vi "Log Message with Level.vi"(6 "Log Level (INFO)":T1=enum."INFO", 8 "error in (no error)":errorcluster, 11 "Message":string) -> (0 "error out":errorcluster)   [LabVIEW 2020, in "RxnRover.lvlib" / "logging.lvlib"]
doc: "Log the given message to the Rxn Rover log file. Appends the log level, date, and time to the message."
uses:
  logging.lvlib
  Log Levels.ctl
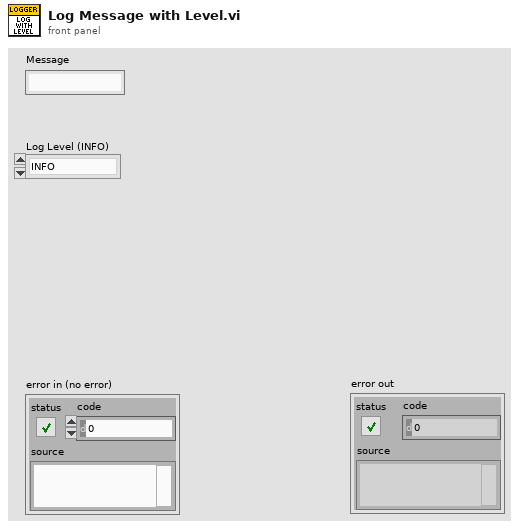
[diagram p1: front panel]
types:
  T1 = typedef "RxnRover.lvlib/logging.lvlib/Log Levels.ctl" = enum16{"NOTSET", "DEBUG", "INFO", "WARNING", "ERROR", "CRITICAL"}
  T2 = typedef "RxnRover.lvlib/logging.lvlib/Log Config.ctl" = cluster{"Log Level":T1}
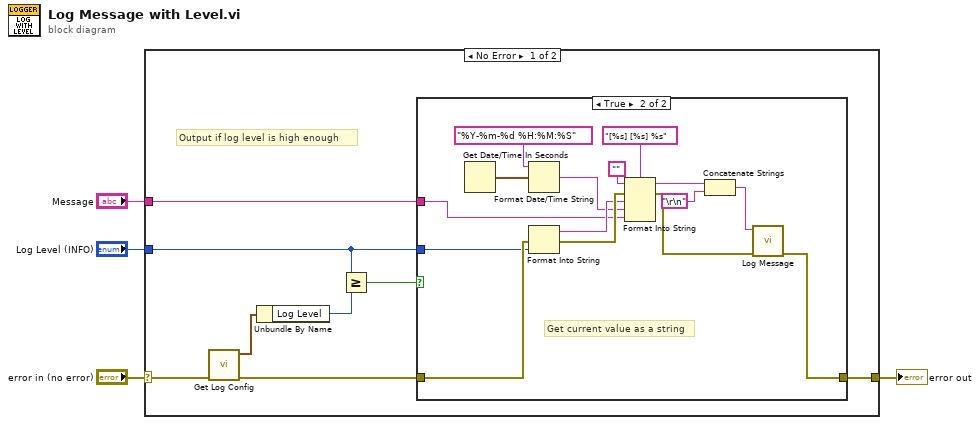
[diagram p0: block diagram]
diagram:
  n1 = case shown="No Error" "error in (no error)" {
    selector: "error in (no error)" -> [w10 w29]
    tunnel: [w12 w29] -> w3
    tunnel: "Log Level (INFO)" -> [w6 _]
    tunnel: "Message" -> [w11 _]
    frame No Error {
      # "Output if log level is high enough"
      n2 = call "Get Log Config.vi"("error in (no error)"=w10) -> ("error out"=w9:errorcluster, "Log Config"=w8:T2)  [unwired: 9 in]
      n3 = Unbundle By Name(w8) -> ("Log Level"=w7:T1)
      n4 = Greater Or Equal?(x=w6, y=w7) -> (x >= y?=w5:bool)
      n5 = case shown="True" w5 {
        tunnel: [w13 w28] -> w12
        tunnel: w11 -> [_ w23]
        tunnel: w9 -> [w13 w15]
        tunnel: w6 -> [_ w14]
        frame False {
        }
        frame True {
          # "Get current value as a string"
          n6 = Get Date/Time In Seconds() -> (seconds since 1Jan1904=w22:timestamp)
          n7 = Format Date/Time String(time format string (%c)="%Y-%m-%d %H:%M:%S", seconds (now)=w22) -> (date/time string=w21:string)  [unwired: 1 in]
          n8 = Format Into String(error in=w15, w14) -> (resulting string=w24:string, error out=w26:errorcluster)  [unwired: 2 in]
          n9 = Format Into String(format string="[%s] [%s] %s", initial string="", error in=w26, w24, w21, w23) -> (resulting string=w20:string, error out=w25:errorcluster)
          n10 = Concatenate Strings(w20, "\r\n") -> (w18:string)
          n11 = call "Log Message.vi"("error in (no error)"=w25, "Message to Log"=w18) -> ("error out"=w28:errorcluster)  [unwired: 9 in]
        }
      }
    }
    frame Error {
    }
  }
  "error out" <- w3
